vi "Actuators Halt.vi"(0 "Notifier Name":string, 11 "Error In":errorcluster) -> (4 "Notifier Name Out":string, 15 "Error Out":errorcluster)   [LabVIEW 2025]
uses:
  Actuators Controls/Actuators Note Type.ctl
  Actuators Controls/Actuators Actions.ctl
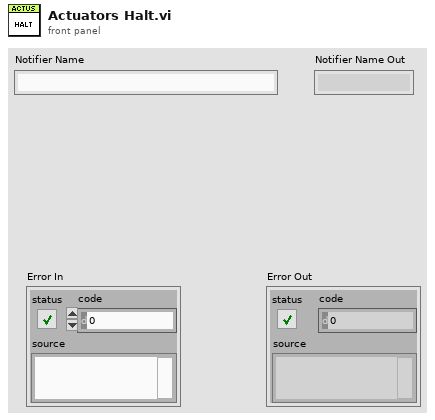
[diagram p1: front panel]
types:
  T1 = typedef "Actuators Note Type.ctl" = cluster{"Actions":T2, "Cmd Received ":bool, "Setpoint":dbl[], "Position":dbl[], "Channel":i32[], "Jog Step":dbl[], "Velocity":dbl[], "Acceleration":dbl[], "Status Bits":u32[], "Moving":bool[]}
  T2 = typedef "Actuators Actions.ctl" = enum16{"Nothing", "Get Position", "Get Acceleration", "Get Velocity", "Get Jog Step", "Set Acceleration", "Set Velocity", "Set Jog Step", "Move Absolute", "Move Relative", "Jog Forward", "Jog Reverse", "Set Moving", "Halt", "Quit"}
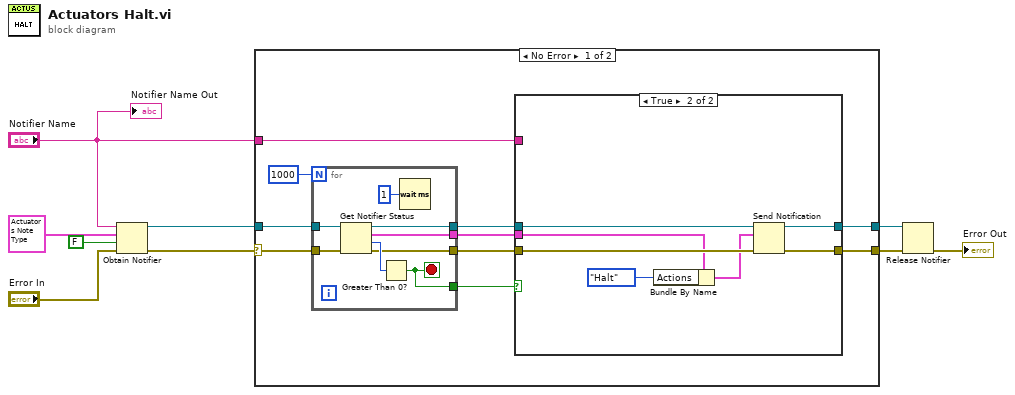
[diagram p0: block diagram]
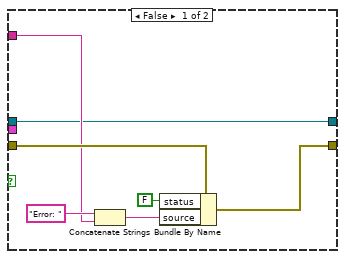
[diagram p2: hidden frame]
diagram:
  n1 = Obtain Notifier(name (unnamed)="Notifier Name", notification data type=T1 {"Actions"=enum."Nothing", "Cmd Received "=FALSE, "Setpoint"=[], "Position"=[], "Channel"=[], "Jog Step"=[], "Velocity"=[], "Acceleration"=[], "Status Bits"=[], "Moving"=[]} ("Actuators Note"), create if not found? (T)=FALSE, error in (no error)="Error In") -> (notifier out=w5:refnum<notifier>, error out=w8:errorcluster)  [unwired: 1 out]
  n2 = case shown="No Error" w8 {
    selector: w8 -> [w17 w42]
    tunnel: w5 -> [w18 w43]
    tunnel: "Notifier Name" -> [w13 _]
    tunnel: [w12 w43] -> w4
    tunnel: [w11 w42] -> w3
    frame No Error {
      n3 = for {
        N: 1000 -> [_]
        tunnel: [w40] -> w15
        tunnel: w18 -> [w41]
        tunnel: [w39] -> w16
        tunnel: w17 -> [w36]
        tunnel: [w35] -> w10
        tunnel: [w34] -> w14
        stop <- w35 stop-if-true
        n4 = Get Notifier Status(notifier=w41, error in (no error)=w36) -> (notifier out=w39:refnum<notifier>, current notification=w40:T1, # waiting=w38:i32, error out=w34:errorcluster)  [unwired: 1 out]
        n5 = Greater Than 0?(x=w38) -> (x > 0?=w35:bool)
        n6 = Wait (ms)(milliseconds to wait=u32 1) -> ()  [unwired: 1 out]
      }
      n7 = case shown="True" w10 {
        tunnel: w16 -> [w21 w33]
        tunnel: w15 -> [_ w29]
        tunnel: w14 -> [w26 w32]
        tunnel: w13 -> [w22 _]
        tunnel: [w21 w28] -> w12
        tunnel: [w20 w27] -> w11
        frame False {
          n8 = Concatenate Strings("Error: " ("source"), w22) -> (w23:string)
          n9 = Bundle By Name(cluster=w26, "status"=FALSE, "source"=w23) -> (w20:errorcluster)
        }
        frame True {
          n10 = Bundle By Name(cluster=w29, "Actions"=Actuators_Actions."Halt") -> (w30:T1)
          n11 = Send Notification(notification=w30, notifier=w33, error in (no error)=w32) -> (notifier out=w28:refnum<notifier>, error out=w27:errorcluster)
        }
      }
    }
    frame Error {
    }
  }
  n12 = Release Notifier(notifier=w4, error in (no error)=w3) -> (error out=→"Error Out":errorcluster)  [unwired: 1 in, 2 out]
  "Notifier Name Out" <- "Notifier Name"
